vi "Tosca-Init Masker Hardware.vi"(0 "Channel":string, 11 "error in (no error)":errorcluster, 12 "Sampling rate (Hz)":dbl=1000.0 format="%0.2f", 13 "Npts":i32) -> (4 "task out":refnum<k21>, 15 "error out":errorcluster)   [LabVIEW 2020]
uses:
  <vilib>/DAQmx/create/channels.llb/DAQmx Create Channel (AO-Voltage-Basic).vi
  <vilib>/DAQmx/configure/timing.llb/DAQmx Timing (Sample Clock).vi
  <resource>/objmgr/daqmx.rc
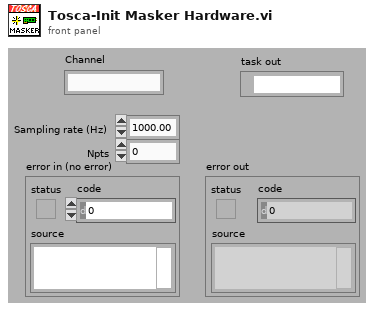
[diagram p1: front panel]
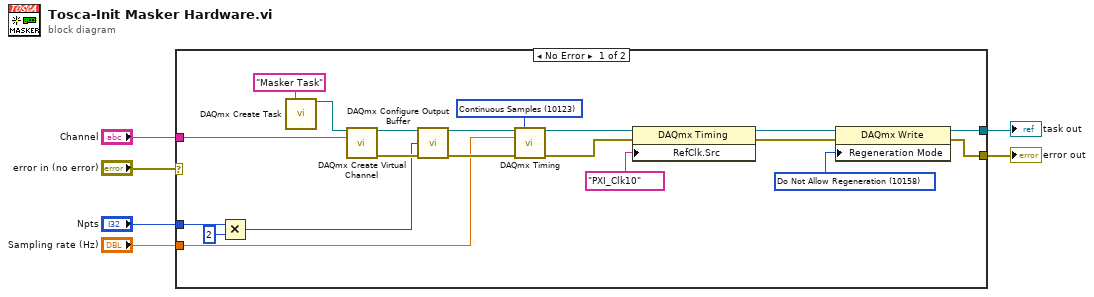
[diagram p0: block diagram]
diagram:
  n1 = case shown="No Error" "error in (no error)" {
    selector: "error in (no error)" -> [_ w27]
    tunnel: "Sampling rate (Hz)" -> [w21 _]
    tunnel: "Npts" -> [w20 _]
    tunnel: "Channel" -> [w7 _]
    tunnel: [w16 _] -> w3
    tunnel: [w15 w27] -> w2
    frame No Error {
      w17 = 10158 items=["Allow Regeneration"=10097, "Do Not Allow Regeneration"=10158] ("RegenMode")
      w22 = 10123 items=["Finite Samples"=10178, "Continuous Samples"=10123, "Hardware Timed Single Point"=12522] ("sample mode")
      n2 = Multiply(x=w20, y=u32 2) -> (x*y=w19:u32)
      n3 = call <vilib>:"DAQmx Create Task.vi"("new task name"="Masker Task") -> ("task out"=w13:refnum<k21>)  [unwired: 13 in, 1 out]
      n4 = call-poly <vilib>:"DAQmx Create Virtual Channel.vi"("task in"=w13, "physical channels"=w7) -> ("task out"=w26:refnum<k21>, "error out"=w23:errorcluster)  [unwired: 12 in]
      n5 = call <vilib>:"DAQmx Configure Output Buffer.vi"("task/channels in"=w26, "buffer size (in samples per channel)"=w19, "error in"=w23) -> ("task out"=w25:refnum<k21>, "error out"=w24:errorcluster)  [unwired: 11 in]
      n6 = call-poly <vilib>:"DAQmx Timing.vi"("task/channels in"=w25, "sample mode"=w22, "rate"=w21, "error in"=w24) -> ("task out"=w11:refnum<k21>, "error out"=w10:errorcluster)  [unwired: 10 in]
      n7 = property class="DAQmx Timing"(reference=w11, error in=w10, "RefClk.Src"=tag "PXI_Clk10") -> (reference out=w9:refnum<k21>, error out=w8:errorcluster)
      n8 = property class="DAQmx Write"(reference=w9, error in=w8, "Regeneration Mode"=w17) -> (reference out=w16:refnum<k21>, error out=w15:errorcluster)
    }
    frame Error {
    }
  }
  "error out" <- w2
  "task out" <- w3
